vi "Set State and Measure Resitance.vi"(6 "SMU Settings":T2={"Level"=0.01, "Level Range"=0.1, "Limit"=1.0, "Limit Range"=6.0, "Sense"=1009} {"Sense" items=["Local"=1008, "Remote"=1009]}, 7 "script name":string, 8 "error in (no error)":errorcluster, 10 "Pins":string[](array[string])=["VDD"], 11 "Semiconductor Module Context":T3) -> (0 "error Out":errorcluster)   [LabVIEW 2013]
uses:
  <vilib>/NI_TestStand_SemiconductorModule/NI_TestStand_Semiconductor_Module.lvlibp/PinMap/General/SemiconductorModuleContext.ctl
  <instrlib>/niDCPower/nidcpower.llb/niDCPower Sense.ctl
  <instrlib>/niHSDIO/niHSDIO.llb/niHSDIO_ctl Trigger Script - trigID Values (Ring).ctl
  <vilib>/NI_TestStand_SemiconductorModule/NI_TestStand_Semiconductor_Module.lvlibp
panel:
  in  "Number_of_Bits":u32=7
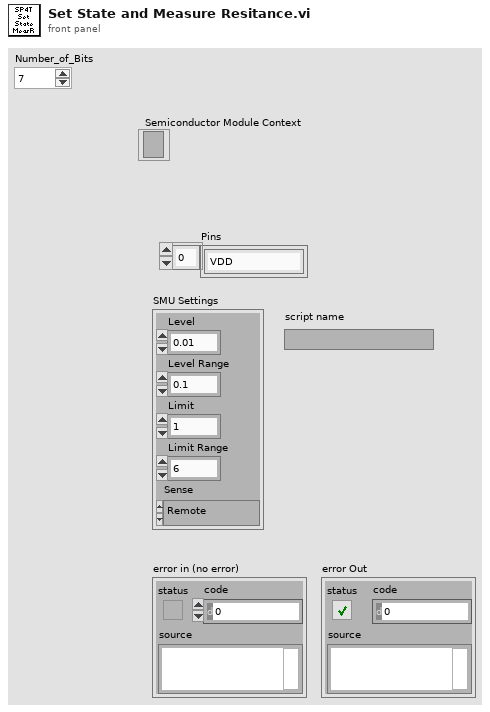
[diagram p1: front panel]
types:
  T1 = typedef "niDCPower Sense.ctl" = i32
  T2 = cluster{"Level":dbl, "Level Range":dbl, "Limit":dbl, "Limit Range":dbl, "Sense":T1}
  T3 = typedef "NI_TestStand_Semiconductor_Module.lvlibp/SemiconductorModuleContext.ctl" = refnum<k7>
  T4 = typedef "niHSDIO_ctl Trigger Script - trigID Values (Ring).ctl" = string
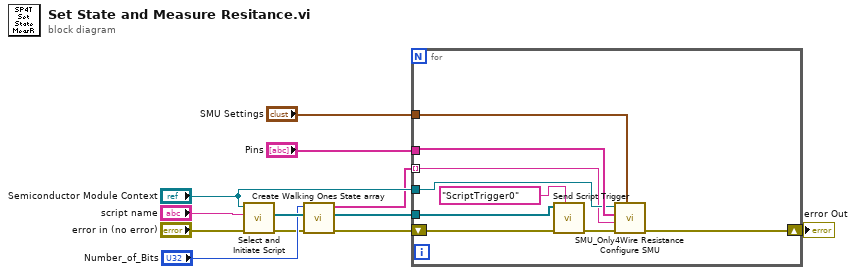
[diagram p0: block diagram]
diagram:
  n1 = call "Select and Initiate Script.vi"("error in (no error)"="error in (no error)", "script name"="script name", "Semiconductor Module Context"="Semiconductor Module Context") -> ("error out"=w3:errorcluster, "HSDIO GEN Sessions Out"=w7:refnum<k15>[])  [unwired: 6 in, 1 out]
  n2 = call "Create Walking Ones State array.vi"("Error In"=w3, "Number_of_Bits"="Number_of_Bits") -> ("Error Out"=w2:errorcluster, "Array"=w1:string[])  [unwired: 8 in]
  n3 = for {
    tunnel: "Semiconductor Module Context" -> [w16]
    tunnel: "Pins" -> [w17]
    shift-right: [w14] -> w10
    shift-left: w2 -> [w20]
    tunnel: w7 -> [w19]
    tunnel: "SMU Settings" -> [w13]
    tunnel: w1 -> [w12] mode=indexing
    n4 = call "Send Script Trigger.vi"("trigger id (script trigger 0)"=T4 "ScriptTrigger0", "error in (no error)"=w20, "HSDIO Sessions In"=w19) -> ("error out"=w15:errorcluster)  [unwired: 7 in, 1 out]
    n5 = call "SMU_Only4Wire Resistance Configure SMU.vi"("SMU Settings"=w13, "error in (no error)"=w15, "Published Data Id"=w12, "Pins"=w17, "Semiconductor Module Context"=w16) -> ("error Out"=w14:errorcluster)  [unwired: 4 in, 2 out]
  }
  "error Out" <- w10
